vi "Is File In LLB.vi"(4 "Path":path) -> (6 "LLB Name":string, 7 "Is in LLB?":bool)   [LabVIEW 2023, in "VIDoc Parsing.lvlib" / "VIDoc Parser.lvclass"]
uses:
  VIDoc Parser.lvclass
  VIDoc Parser.lvclass/VIDoc Parser.ctl
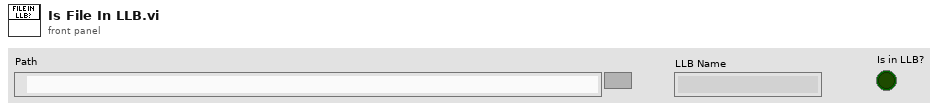
[diagram p1: front panel]
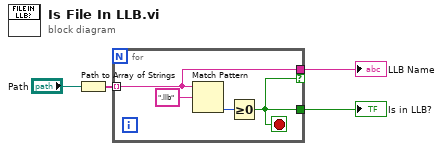
[diagram p0: block diagram]
diagram:
  n1 = Path to Array of Strings(0:"Path") -> (2:w2:string[])  [unwired: 1 out]
  n2 = for {
    tunnel: [w5] -> w4
    tunnel: w2 -> [w6] mode=indexing
    tunnel: [w6] -> w1 if=w5
    stop <- w5 stop-if-true
    n3 = Match Pattern(string=w6, regular expression=".llb") -> (offset past match=w7:i32)  [unwired: 1 in, 3 out]
    n4 = Greater Or Equal To 0?(x=w7) -> (x >= 0?=w5:bool)
  }
  "Is in LLB?" <- w4
  "LLB Name" <- w1
